vi "FindIntersectionOfRectangles.vi"(10 "Wire":T2, 11 "Node Pos":T1) -> (3 "Intersecting?":bool)   [LabVIEW 2014]
uses:
  <vilib>/Utility/miscctls.llb/LVRectTypeDef.ctl
  <vilib>/Utility/miscctls.llb/LVPositionTypeDef.ctl
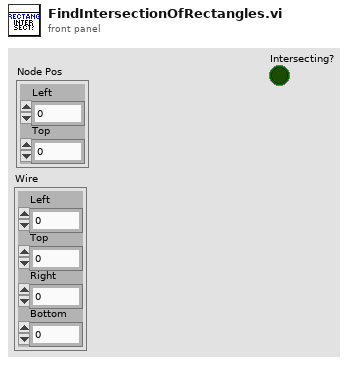
[diagram p1: front panel]
types:
  T1 = typedef "LVPositionTypeDef.ctl" = cluster{"Left":i32, "Top":i32}
  T2 = typedef "LVRectTypeDef.ctl" = cluster{"Left":i16, "Top":i16, "Right":i16, "Bottom":i16}
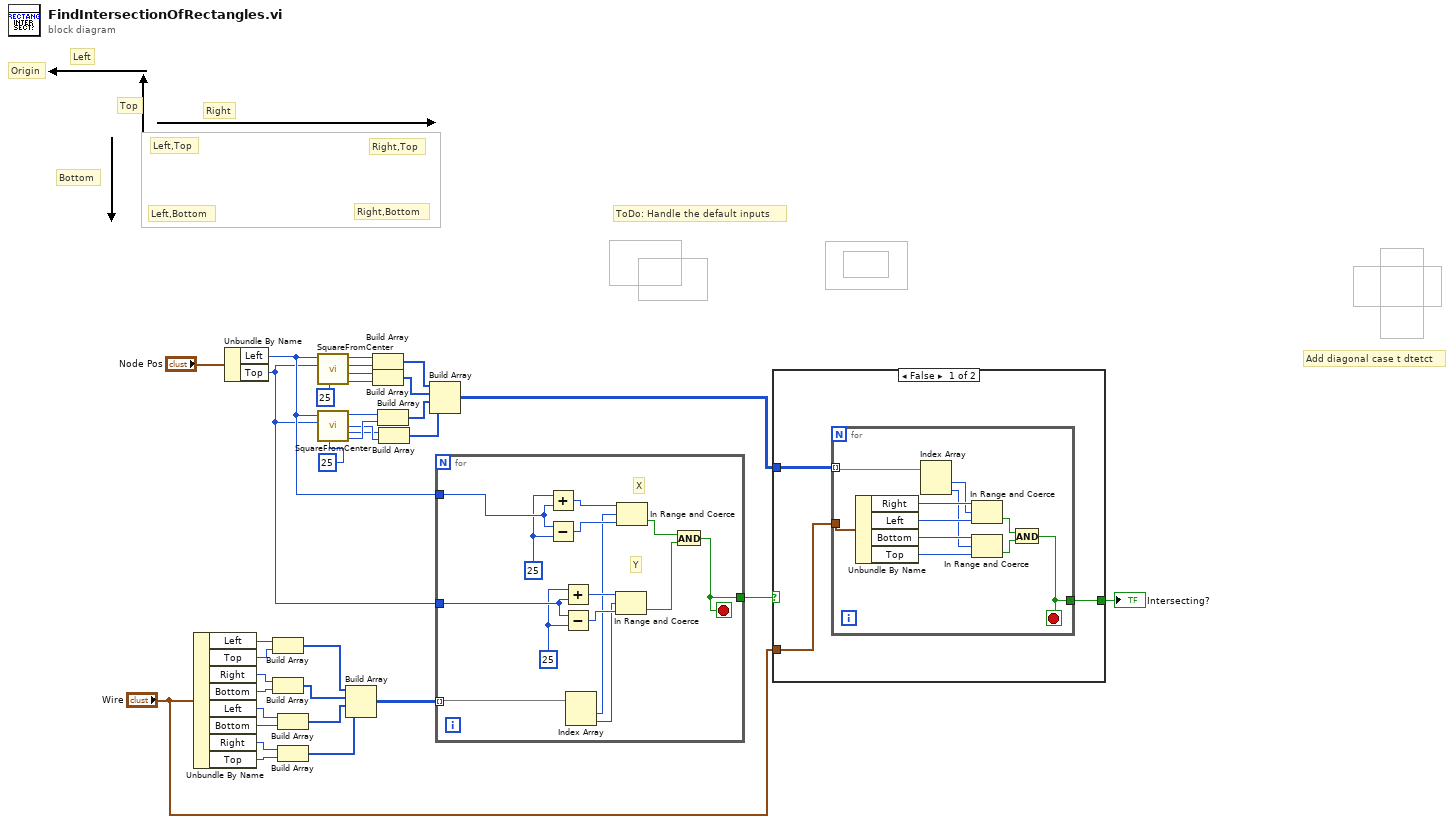
[diagram p0: block diagram]
diagram:
  # "ToDo: Handle the default inputs"
  # "Add diagonal case t dtetct"
  # "Bottom"
  # "Right"
  # "Left,Bottom"
  # "Right,Bottom"
  # "Right,Top"
  # "Left,Top"
  # "Top"
  # "Origin"
  # "Left"
  n1 = Unbundle By Name("Wire") -> ("Left"=w30:i16, "Top"=w29:i16, "Right"=w28:i16, "Bottom"=w27:i16, "Left"=w25:i16, "Bottom"=w26:i16, "Right"=w24:i16, "Top"=w23:i16)
  n2 = Unbundle By Name("Node Pos") -> ("Left"=w9:i32, "Top"=w8:i32)
  n3 = Build Array(w30, w29) -> (w22:i16[])
  n4 = Build Array(w28, w27) -> (w21:i16[])
  n5 = Build Array(w25, w26) -> (w20:i16[])
  n6 = Build Array(w24, w23) -> (w19:i16[])
  n7 = call "SquareFromCenter.vi"("Distance"=25, "Top"=w8, "Left"=w9) -> ("Bottom"=w10:i32, "Right"=w11:i32, "Top 2"=w12:i32, "Left 2"=w13:i32)  [unwired: 5 in]
  n8 = call "SquareFromCenter.vi"("Distance"=25, "Top"=w8, "Left"=w9) -> ("Bottom"=w6:i32, "Right"=w4:i32, "Top 2"=w5:i32, "Left 2"=w7:i32)  [unwired: 5 in]
  n9 = Build Array(w22, w21, w20, w19) -> (w18:i16[][])
  n10 = Build Array(w13, w12) -> (w14:i32[])
  n11 = Build Array(w11, w10) -> (w15:i32[])
  n12 = Build Array(w7, w6) -> (w16:i32[])
  n13 = Build Array(w4, w5) -> (w17:i32[])
  n14 = Build Array(w14, w15, w16, w17) -> (w3:i32[][])
  n15 = for {
    tunnel: [w48] -> w33
    tunnel: w9 -> [w47]
    tunnel: w8 -> [w46]
    tunnel: w18 -> [w39] mode=indexing
    stop <- w48 stop-if-true
    w42 = 25 ("Left")
    w43 = 25 ("Left")
    # "Y"
    # "X"
    n16 = Add(x=w43, y=w47) -> (x+y=w44:i32)
    n17 = Subtract(x=w47, y=w43) -> (x-y=w45:i32)
    n18 = Add(x=w42, y=w46) -> (x+y=w41:i32)
    n19 = Subtract(x=w46, y=w42) -> (x-y=w40:i32)
    n20 = Index Array(array=w39) -> (element #1=w38:i16, element #2=w37:i16)  [unwired: 2 in]
    n21 = In Range and Coerce(upper limit=w41, x=w37, lower limit=w40) -> (In Range?=w35:bool)  [unwired: 1 out]
    n22 = In Range and Coerce(upper limit=w44, x=w38, lower limit=w45) -> (In Range?=w36:bool)  [unwired: 1 out]
    n23 = And(x=w36, y=w35) -> (x .and. y?=w48:bool)
  }
  n24 = case shown="False" w33 {
    selector: w33 -> [_ w63]
    tunnel: "Wire" -> [w51 _]
    tunnel: [w50 w63] -> w32
    tunnel: w3 -> [w49 _]
    frame False {
      n25 = for {
        tunnel: w51 -> [w59]
        tunnel: [w62] -> w50
        tunnel: w49 -> [w54] mode=indexing
        stop <- w62 stop-if-true
        n26 = Unbundle By Name(w59) -> ("Right"=w58:i16, "Left"=w57:i16, "Bottom"=w56:i16, "Top"=w55:i16)
        n27 = Index Array(array=w54) -> (element #1=w53:i32, element #2=w52:i32)  [unwired: 2 in]
        n28 = In Range and Coerce(upper limit=w58, x=w53, lower limit=w57) -> (In Range?=w61:bool)  [unwired: 1 out]
        n29 = In Range and Coerce(upper limit=w56, x=w52, lower limit=w55) -> (In Range?=w60:bool)  [unwired: 1 out]
        n30 = And(x=w61, y=w60) -> (x .and. y?=w62:bool)
      }
    }
    frame True {
    }
  }
  "Intersecting?" <- w32
